vi "cmd status.vi"(8 "error in (no error)":errorcluster, 11 "motor in":refnum<class "AISAS motor.lvclass">) -> (0 "error out":errorcluster, 2 "Motor status":T1, 3 "motor out":refnum<class "AISAS motor.lvclass">, 5 "Motor Ok?":bool, 7 "status log":string)   [LabVIEW 2014, in "AISAS motor.lvclass"]
uses:
  AISAS motor.lvclass
  Controls/motor.ctl
  Motor status.ctl
  AISAS motor.lvclass/AISAS motor.ctl
panel:
  out "Motor":T2
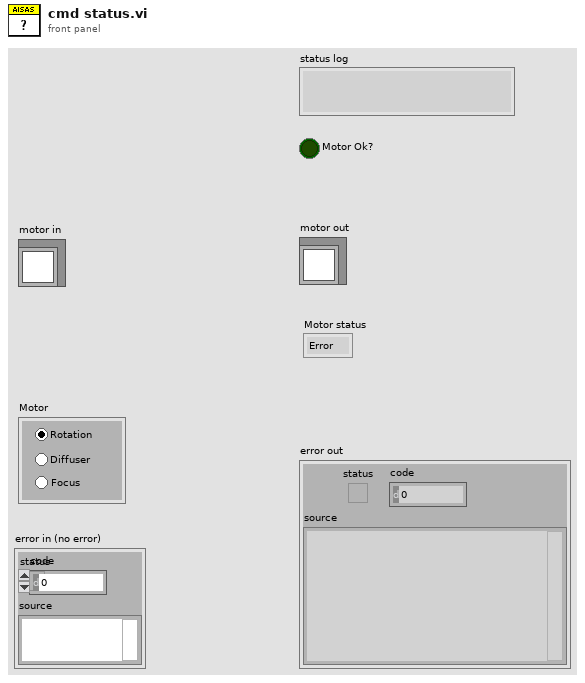
[diagram p1: front panel]
types:
  T1 = typedef "AISAS motor.lvclass/Motor status.ctl" = enum16{"Error", "Ready", "Bussy"}
  T2 = typedef "motor.ctl" = enum32{"Rotation", "Diffuser ", "Focus"}
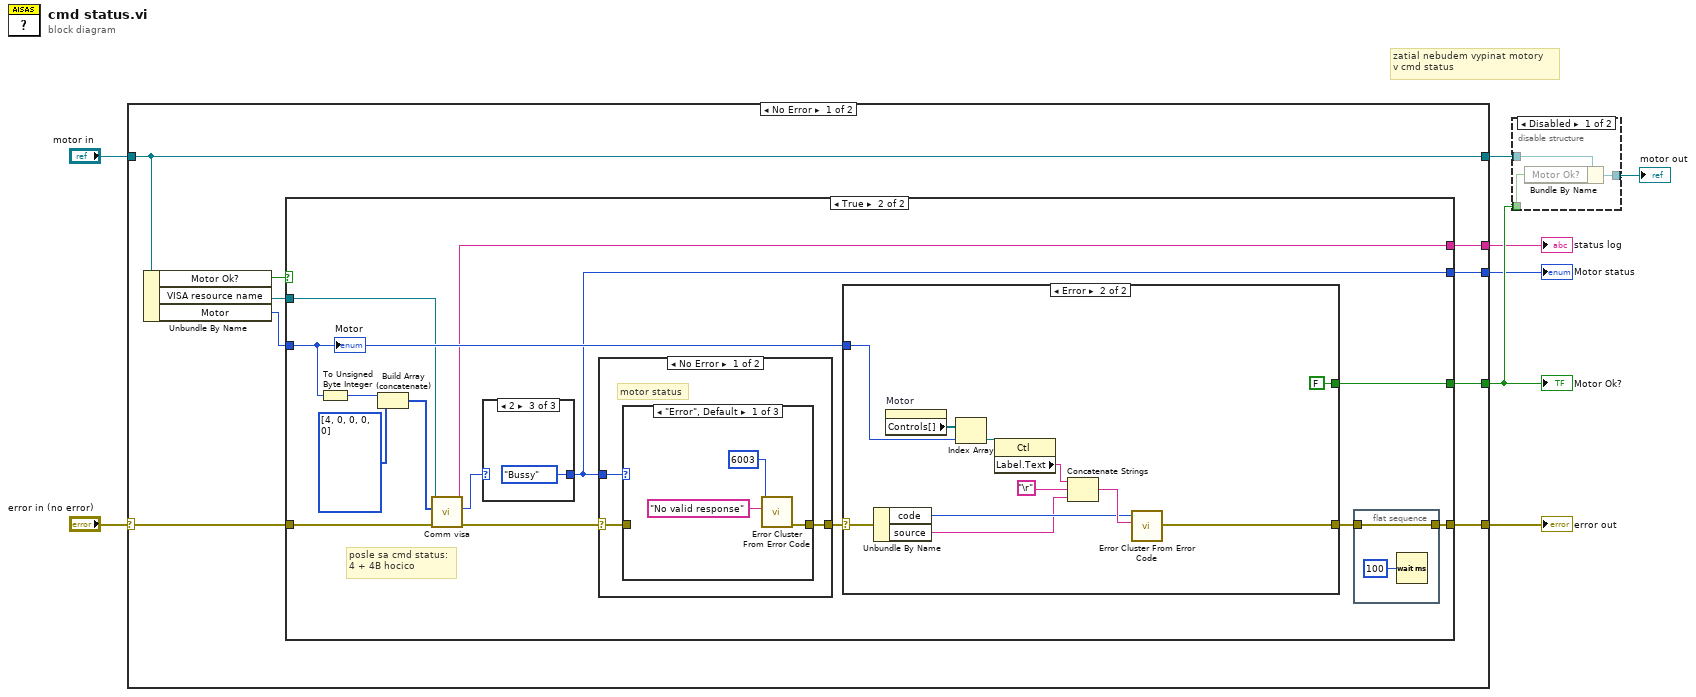
[diagram p0: block diagram]
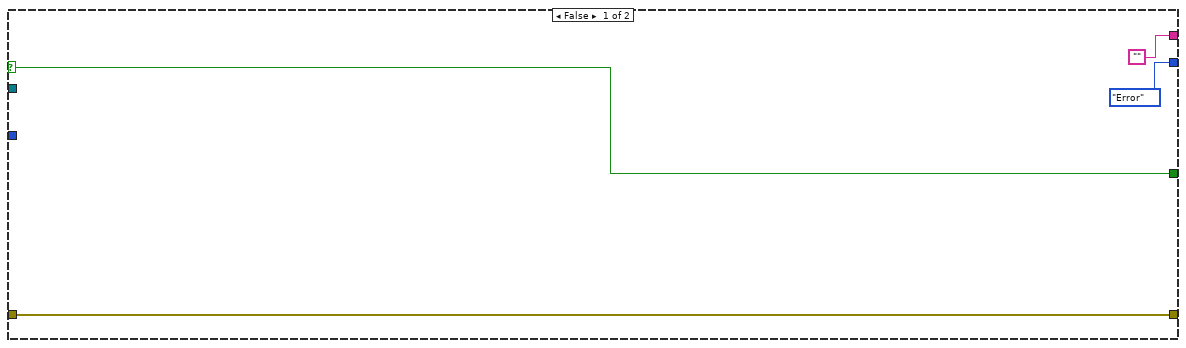
[diagram p3: hidden frame]
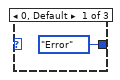
[diagram p4: hidden frame]
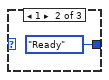
[diagram p5: hidden frame]
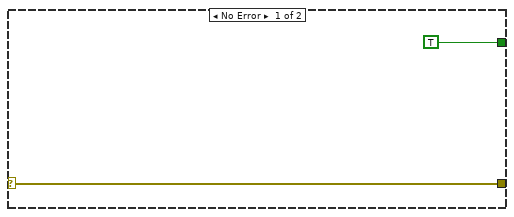
[diagram p6: hidden frame]
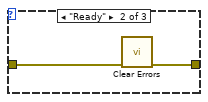
[diagram p7: hidden frame]
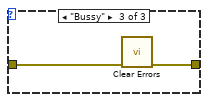
[diagram p8: hidden frame]
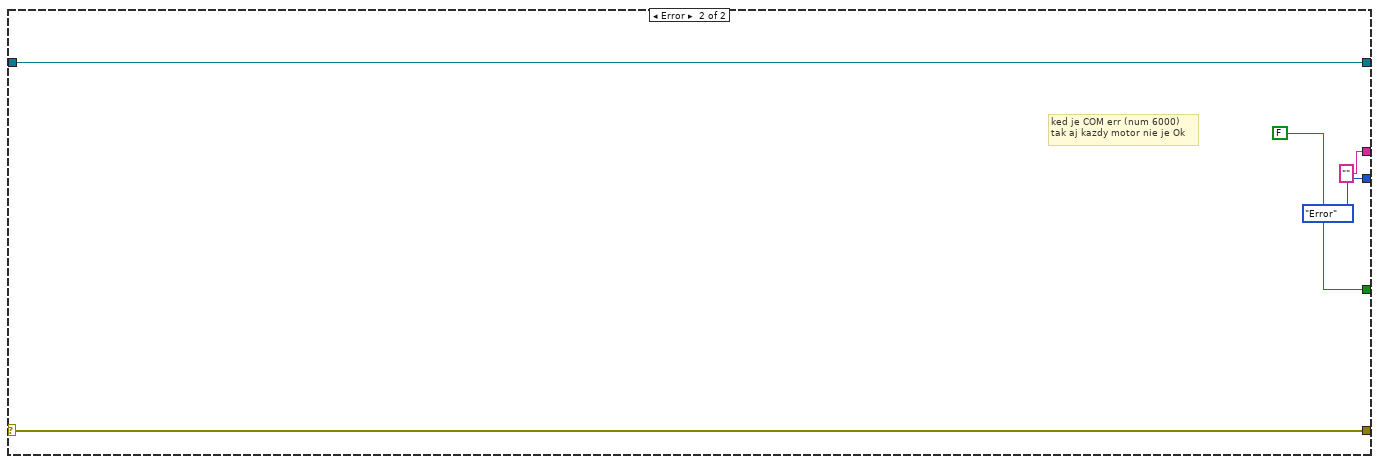
[diagram p10: hidden frame]
diagram:
  # "zatial nebudem vypinat motory\nv cmd status"
  n1 = case shown="No Error" "error in (no error)" {
    selector: "error in (no error)" -> [w16 w69]
    tunnel: [w17 w69] -> w7
    tunnel: "motor in" -> [w14 w68]
    tunnel: [w15 FALSE ("Motor Ok")] -> w5
    tunnel: [w14 w68] -> w4
    tunnel: [w12 "" ("Log response")] -> w2
    tunnel: [w9 Motor_status."Error" ("Motor status")] -> w1
    frame No Error {
      n2 = Unbundle By Name(w14) -> ("Motor Ok?"=w11:bool, "VISA resource name"=w13:refnum<visa-resource-name>, "Motor"=w10:T2)
      n3 = case shown="True" w11 {
        selector: w11 -> [w19 _]
        tunnel: [w19 w34] -> w15
        tunnel: [w21 w25] -> w17
        tunnel: w10 -> [_ w32]
        tunnel: w16 -> [w21 w31]
        tunnel: ["" w27] -> w12
        tunnel: w13 -> [_ w22]
        tunnel: [Motor_status."Error" ("Motor status") w23] -> w9
        frame False {
        }
        frame True {
          # "posle sa cmd status:\n4 + 4B hocico"
          n4 = To Unsigned Byte Integer(number=w32) -> (unsigned 8bit integer=w30:u8)
          n5 = Build Array (concatenate)(w30, u8[] [4, 0, 0, 0, 0]) -> (w28:u8[])
          n6 = call "Comm visa.vi"("error in (no error)"=w31, "Command"=w28, "VISA in"=w22) -> ("error out"=w33:errorcluster, "status log"=w27:string, "Response"=w24:u8)  [unwired: 5 in, 1 out]
          n7 = case shown="2" w24 {
            tunnel: [Motor_status."Error" ("Motor status") Motor_status."Ready" ("Motor status") Motor_status."Bussy" ("Motor status")] -> w23
            frame 0, Default {
            }
            frame 1 {
            }
            frame 2 {
            }
          }
          n8 = case shown="No Error" w33 {
            selector: w33 -> [w56 w64]
            tunnel: [w55 w64] -> w35
            tunnel: w23 -> [w54 _]
            frame No Error {
              # "motor status"
              n9 = case shown="\"Error\", Default" w54 {
                tunnel: w56 -> [_ w61 w63]
                tunnel: [w57 w60 w62] -> w55
                frame "Error", Default {
                  n10 = call <vilib>:"Error Cluster From Error Code.vi"("error message (\"\")"="No valid response" ("error message (\"\")"), "error code (0)"=6003) -> ("error out"=w57:errorcluster)  [unwired: 7 in]
                }
                frame "Ready" {
                  n11 = call <vilib>:"Clear Errors.vi"("error in (no error)"=w61) -> ("error out"=w60:errorcluster)  [unwired: 5 in, 1 out]
                }
                frame "Bussy" {
                  n12 = call <vilib>:"Clear Errors.vi"("error in (no error)"=w63) -> ("error out"=w62:errorcluster)  [unwired: 5 in, 1 out]
                }
              }
            }
            frame Error {
            }
          }
          n13 = case shown="Error" w35 {
            selector: w35 -> [w41 w49]
            tunnel: [TRUE ("Motor Ok") FALSE ("Motor Ok")] -> w34
            tunnel: w32 -> [_ w50]
            tunnel: [w41 w45] -> w26
            frame No Error {
            }
            frame Error {
              n14 = Unbundle By Name(w49) -> ("code"=w47:i32, "source"=w46:string)
              n15 = property on="Motor" class="RadioBtnsControl (strict)"() -> ("Controls[]"=w52:refnum<vi>[])  [unwired: 2 in, 2 out]
              n16 = Index Array(array=w52, index=w50) -> (element=w51:refnum<vi>)
              n17 = property class="Ctl"(reference=w51) -> ("Label.Text"=w44:string)  [unwired: 1 in, 2 out]
              n18 = Concatenate Strings(w44, "\r", w46) -> (w48:string)
              n19 = call <vilib>:"Error Cluster From Error Code.vi"("error message (\"\")"=w48, "error code (0)"=w47) -> ("error out"=w45:errorcluster)  [unwired: 7 in]
            }
          }
          n20 = flat-sequence {
            tunnel: w26 -> [w40]
            tunnel: [w40] -> w25
            frame #0 {
              n21 = Wait (ms)(milliseconds to wait=u32 100) -> ()  [unwired: 1 out]
            }
          }
          "Motor" <- w32
        }
      }
    }
    frame Error {
      # "ked je COM err (num 6000)\ntak aj kazdy motor nie je Ok"
    }
  }
  "error out" <- w7
  "Motor Ok?" <- w5
  "status log" <- w2
  "Motor status" <- w1
  n22 = disable-structure shown="Disabled" {
    disable-tunnel: w5 -> [w72 _]
    disable-tunnel: w4 -> [w71 w73]
    disable-tunnel: [w70 w73] -> w3
    frame Disabled {
      n23 = Bundle By Name(cluster=w71, "Motor Ok?"=w72) -> (w70:refnum<class "AISAS motor.lvclass">)
    }
    frame Enabled {
    }
  }
  "motor out" <- w3
